vi "Read AppBar State.vi"(8 "error in (no error)":errorcluster, 11 "MainController in":refnum<class "MainController.lvclass">) -> (0 "error out":errorcluster, 2 "Enum":T1, 3 "MainController out":refnum<class "MainController.lvclass">)   [LabVIEW 2012, in "Win8uiFramework.lvlib" / "MainController.lvclass"]
uses:
  MainController.lvclass
  Visiblity States.ctl
  MainController.lvclass/MainController.ctl
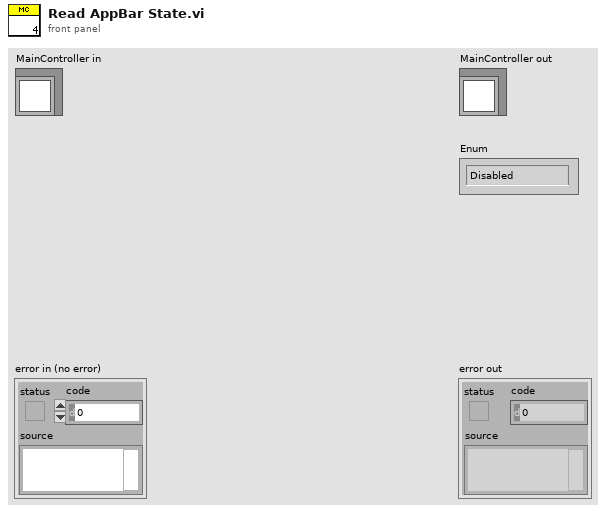
[diagram p1: front panel]
types:
  T1 = typedef "Win8uiFramework.lvlib/MainController.lvclass/Visiblity States.ctl" = enum16{"Disabled", "Hidden - Unpopulated", "Hidden - Populated", "Visible"}
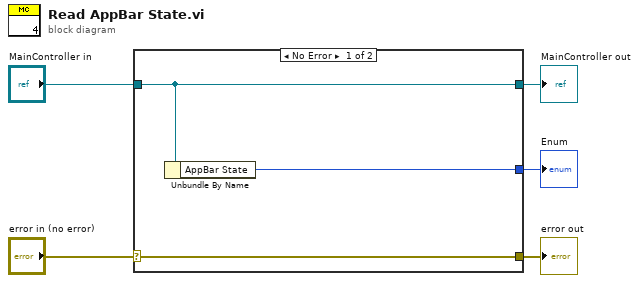
[diagram p0: block diagram]
diagram:
  n1 = case shown="No Error" "error in (no error)" {
    selector: "error in (no error)" -> [w8 w9]
    tunnel: [w8 w9] -> w4
    tunnel: [w7 w10] -> w2
    tunnel: "MainController in" -> [w7 w10]
    tunnel: [w6 _] -> w1
    frame No Error {
      n2 = Unbundle By Name(w7) -> ("AppBar State"=w6:T1)
    }
    frame Error {
    }
  }
  "error out" <- w4
  "MainController out" <- w2
  "Enum" <- w1
